vi "Release-all-client-channels.vi"(8 "error in (no error)":errorcluster, 11 "ModComm in":T1) -> (0 "error out":errorcluster, 3 "ModComm out":T1)   [LabVIEW 2013, in "SLMServer.lvlib" / "SLMServer.lvclass"]
uses:
  SLMServer.lvclass
  Object-reference.ctl
  SLMServer.lvclass/SLMServer.ctl
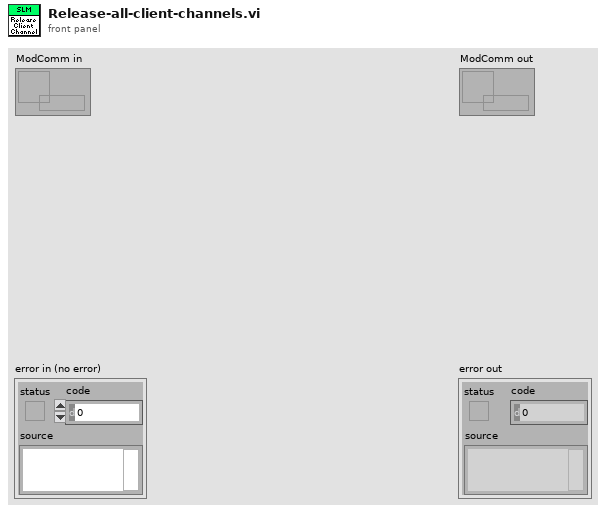
[diagram p1: front panel]
types:
  T1 = typedef "SLMServer.lvlib/SLMServer.lvclass/Object-reference.ctl" = refnum<data-value>
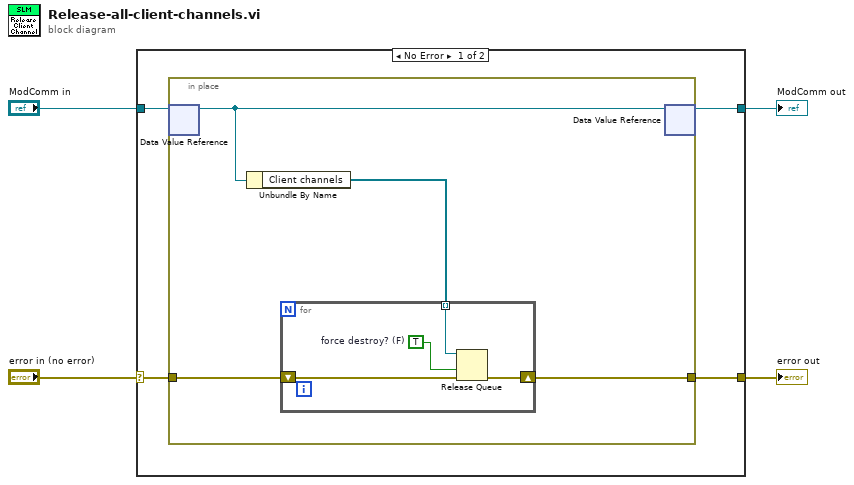
[diagram p0: block diagram]
diagram:
  n1 = case shown="No Error" "error in (no error)" {
    selector: "error in (no error)" -> [w6 w18]
    tunnel: [w5 w18] -> w3
    tunnel: [w7 w17] -> w1
    tunnel: "ModComm in" -> [w8 w17]
    frame No Error {
      n2 = in-place {
        in-place-border: w6 -> [w12]
        in-place-border: [w11] -> w5
        n3 = in-place-dvr #1(w8) -> (w10:refnum<class "SLMServer.lvclass">)  [unwired: 1 out]
        n4 = Unbundle By Name(w10) -> ("Client channels"=w9:refnum<queue>[])
        n5 = for {
          tunnel: w9 -> [w14] mode=indexing
          shift-right: [w15] -> w11
          shift-left: w12 -> [w16]
          w13 = TRUE  # force destroy? (F)
          n6 = Release Queue(queue=w14, force destroy? (F)=w13, error in (no error)=w16) -> (error out=w15:errorcluster)  [unwired: 2 out]
        }
        n7 = in-place-dvr #1(w10) -> (w7:T1)  [unwired: 1 out]
      }
    }
    frame Error {
    }
  }
  "error out" <- w3
  "ModComm out" <- w1
